vi "RSE.vi"(9 "e[n]":dbl, 10 "Numeric":i32, 11 "RSE in":dbl[](array[numeric])) -> (3 "RSE out":dbl[](array[numeric]))   [LabVIEW 2013]
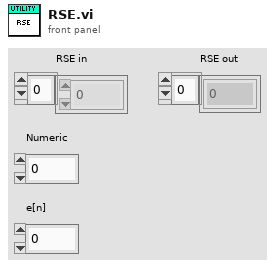
[diagram p1: front panel]
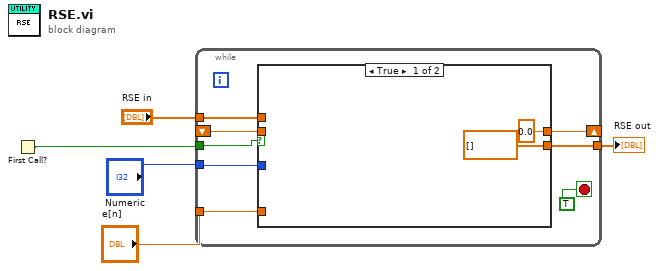
[diagram p0: block diagram]
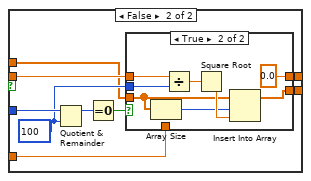
[diagram p2: hidden frame]
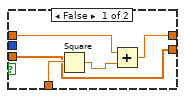
[diagram p3: hidden frame]
diagram:
  n1 = First Call?() -> (First Call?: T/F=w1:bool)
  n2 = while {
    tunnel: "Numeric" -> [w13]
    shift-right: [w9] -> _
    shift-left: _ -> [w10]
    tunnel: "e[n]" -> [w11]
    tunnel: "RSE in" -> [w8]
    tunnel: [w7] -> w5
    tunnel: w1 -> [w6]
    stop <- TRUE stop-if-true
    n3 = case shown="True" w6 {
      tunnel: w13 -> [_ w24]
      tunnel: w11 -> [_ w21]
      tunnel: w10 -> [_ w20]
      tunnel: [0.0 w19] -> w9
      tunnel: w8 -> [_ w17]
      tunnel: [dbl[] [] ("RSE in") w16] -> w7
      frame True {
      }
      frame False {
        w18 = 100 ("y")
        n4 = Quotient & Remainder(x=w24, y=w18) -> (x-y*floor(x/y)=w23:i32)  [unwired: 1 out]
        n5 = Equal To 0?(x=w23) -> (x = 0?=w22:bool)
        n6 = case shown="True" w22 {
          tunnel: w21 -> [w29 _]
          tunnel: w20 -> [w27 w36]
          tunnel: [w26 0.0] -> w19
          tunnel: w18 -> [_ w35]
          tunnel: w17 -> [w25 w31]
          tunnel: [w25 w32] -> w16
          frame False {
            n7 = Square(x=w29) -> (x^2=w28:dbl)
            n8 = Add(x=w27, y=w28) -> (x+y=w26:dbl)
          }
          frame True {
            n9 = Array Size(array=w31) -> (size(s)=w30:i32)
            n10 = Divide(x=w36, y=w35) -> (x/y=w34:dbl)
            n11 = Square Root(x=w34) -> (sqrt(x)=w33:dbl)
            n12 = Insert Into Array(array=w31, index=w30, new element=w33) -> (w32:dbl[])
          }
        }
      }
    }
  }
  "RSE out" <- w5
